vi "Simple Register.vi"(0 "bus data input":u64, 5 "bus address":u8, 9 "bus write pulse":bool, 12 "register offset":u8) -> (4 "bus data output":u64, 10 "register contents":u64)   [LabVIEW 2013, in "DIO SPI User Library.lvlib"]
doc: "Simple 64-bit register implementation"
uses:
  DIO SPI User Library.lvlib
panel:
  # "Simple 64-bit register implementation"
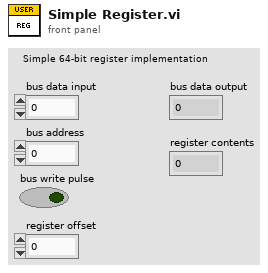
[diagram p1: front panel]
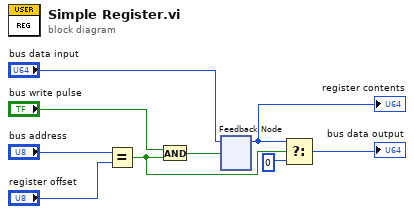
[diagram p0: block diagram]
diagram:
  n1 = Equal?(x="bus address", y="register offset") -> (x = y?=w4:bool)
  n2 = And(x="bus write pulse", y=w4) -> (x .and. y?=w5:bool)
  n3 = feedback #1() -> (w3:u64)  [unwired: 1 in]
  "register contents" <- w3
  n4 = feedback-in #1("bus data input", w5) -> ()
  n5 = Select(t=w3, s=w4, f=u64 0) -> (s? t:f=→"bus data output":u64)
